vi "CloseServo.vi"(8 "error in":errorcluster, 11 "powerServoSession":u32) -> (0 "error out":errorcluster)   [LabVIEW 2016, in "Power Servo.lvlib"]
uses:
  Power Servo.lvlib
  <userlib>/_NI Power Servoing IP/HostRdl/NI Power Servoing IP New (Host).lvlib
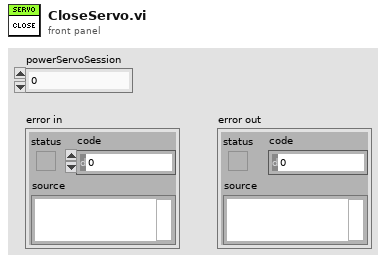
[diagram p1: front panel]
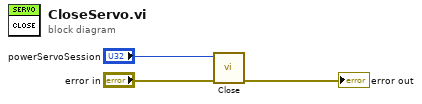
[diagram p0: block diagram]
diagram:
  n1 = call <userlib>:"Close.vi"("error in"="error in", "SessionHandle"="powerServoSession") -> ("error out"=→"error out":errorcluster)  [unwired: 9 in]
